vi "Write Test Progress Msg.vi"(10 "Test.lvlib:Test Progress Msg.lvclass":refnum<class "Test Progress Msg.lvclass">, 11 "Test in":refnum<class "Test.lvclass">) -> (3 "Test out":refnum<class "Test.lvclass">)   [LabVIEW 2017, in "Test.lvlib" / "Test.lvclass"]
uses:
  Test.lvclass
  Test Messages/Test Progress Msg/Test Progress Msg.lvclass
  Test.lvclass/Test.ctl
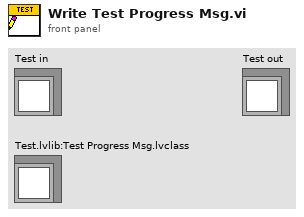
[diagram p1: front panel]
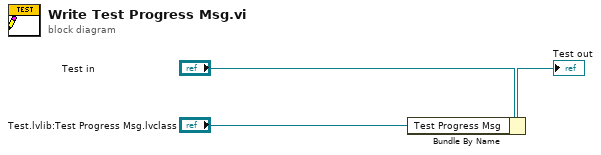
[diagram p0: block diagram]
diagram:
  n1 = Bundle By Name(cluster="Test in", "Test Progress Msg"="Test.lvlib:Test Progress Msg.lvclass") -> (→"Test out":refnum<class "Test.lvclass">)
